vi "CRYRub & Buzz FFT.vi"(11 "wave data":dbl[](array[numeric])) -> (0 "Fe[n,kf]":dbl[][](array[numeric]), 1 "size":i32, 2 "Frame number":i32, 3 "F[k]":dbl[](array[numeric]))   [LabVIEW 2013]
uses:
  <vilib>/Analysis/2dsp.llb/Real FFT.vi
  <vilib>/Analysis/NI_AALPro.lvlib
  <vilib>/measure/NI_MABase.lvlib
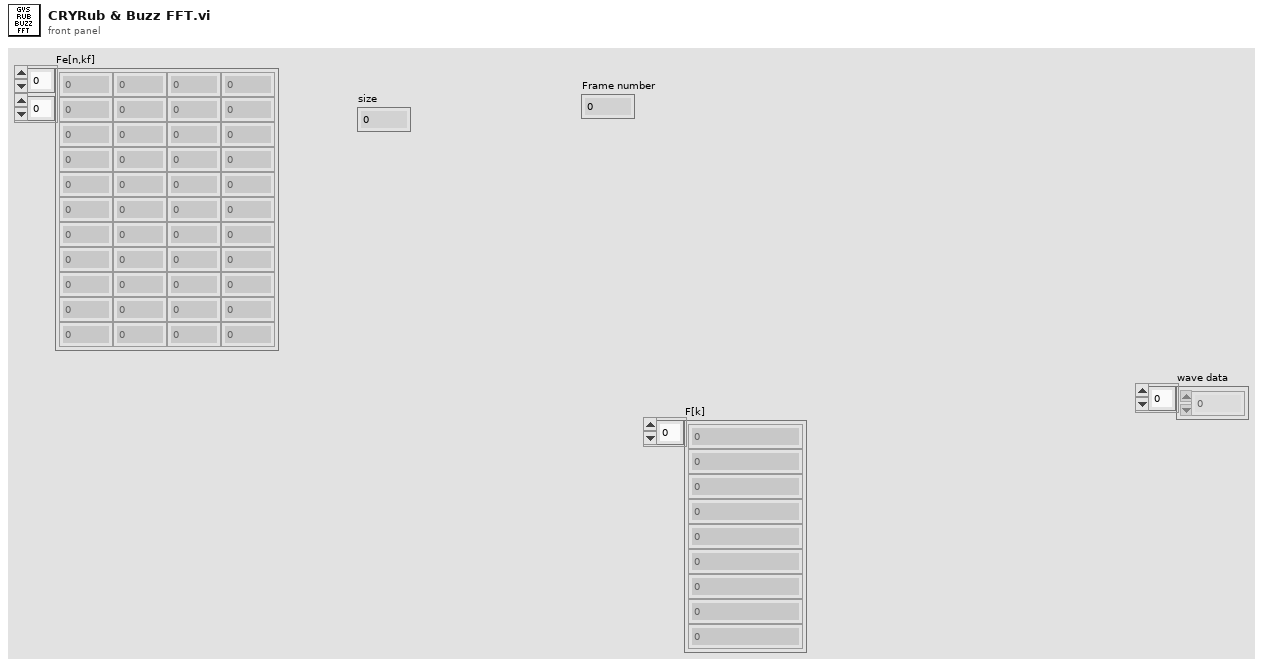
[diagram p1: front panel]
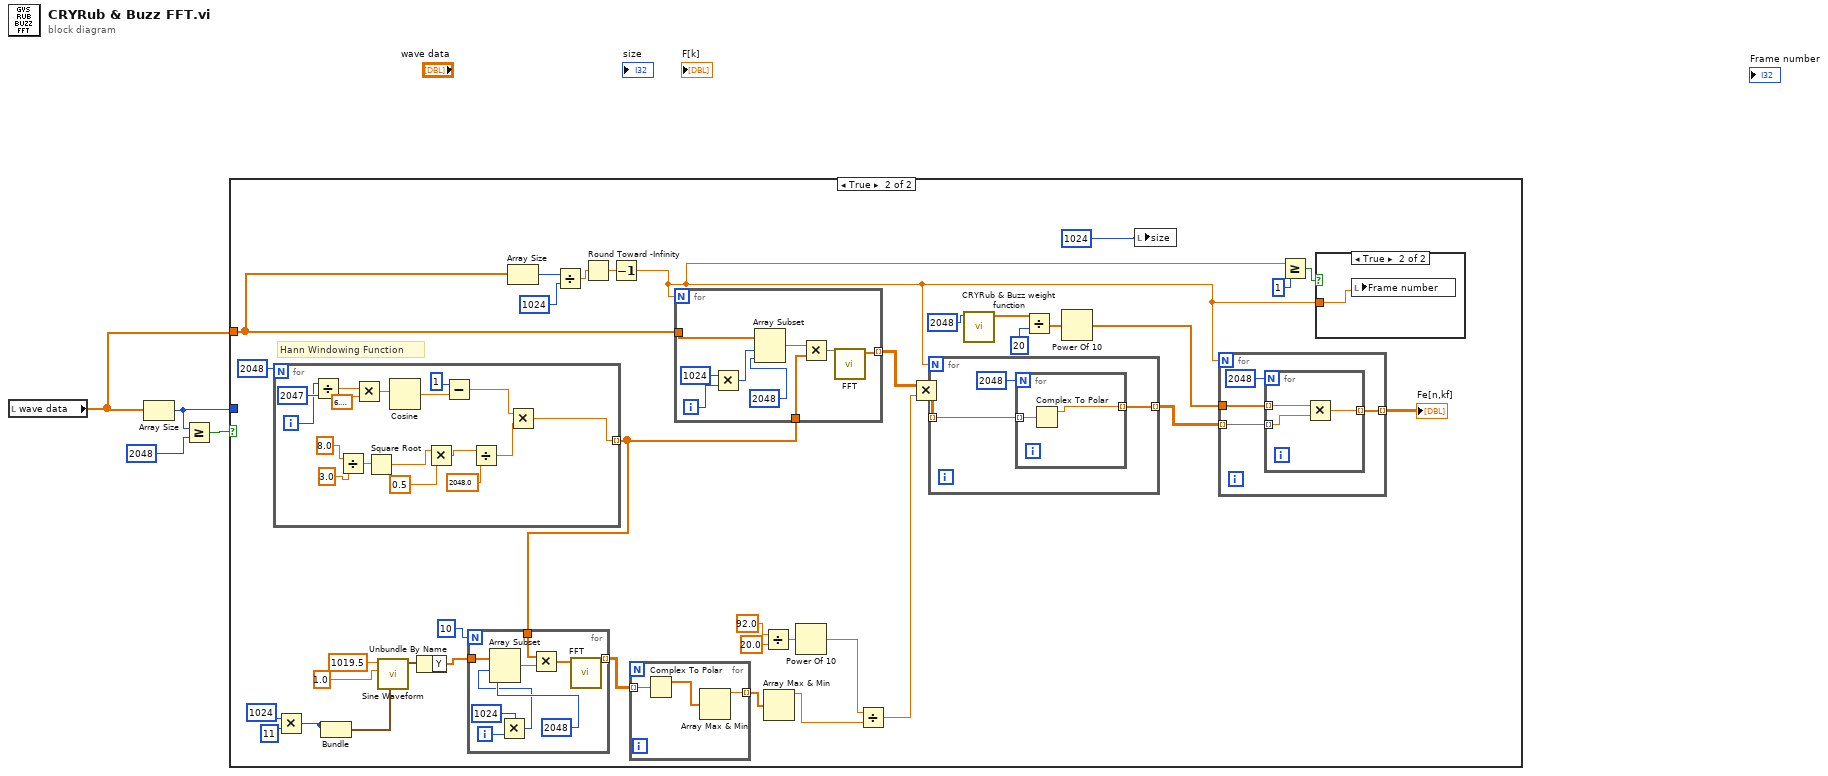
[diagram p0: block diagram]
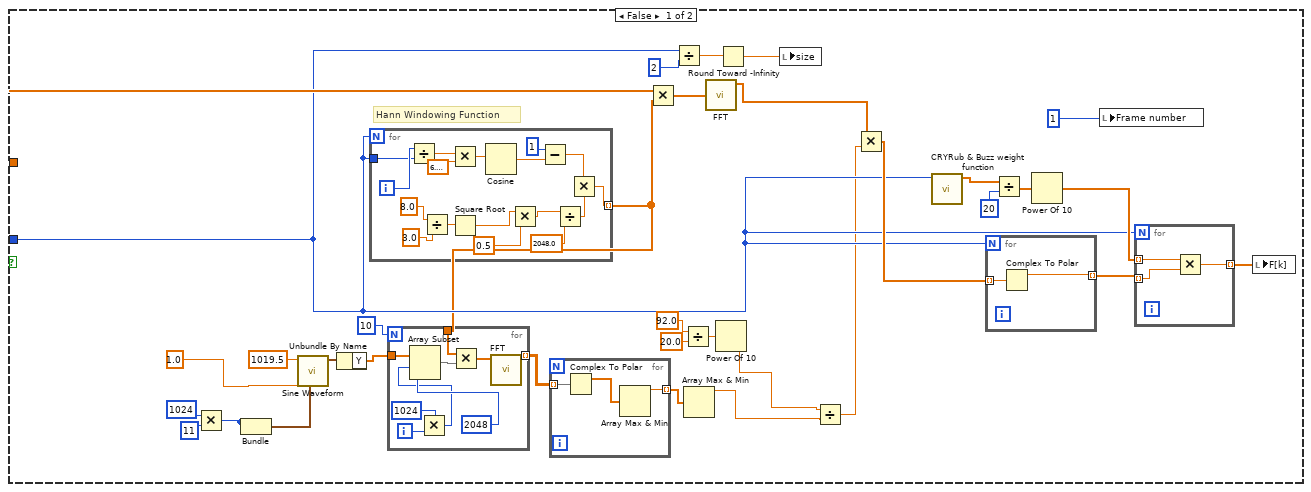
[diagram p2: hidden frame]
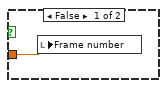
[diagram p3: hidden frame]
diagram:
  n1 = local read "wave data"() -> (w2:dbl[])
  n2 = Array Size(array=w2) -> (size(s)=w1:i32)
  n3 = Greater Or Equal?(x=w1, y=2048) -> (x >= y?=w3:bool)
  n4 = case shown="True" w3 {
    tunnel: w2 -> [w28 w97]
    tunnel: w1 -> [w23 _]
    frame False {
      # "Hann Windowing Function"
      n5 = Multiply(x=1024 ("length"), y=11) -> (x*y=w17:i32)
      n6 = Bundle(w17, w17) -> (w18:cluster{i32, i32})  [unwired: 1 in]
      n7 = call <vilib>:"Sine Waveform.vi"("sampling info"=w18, "amplitude"=1.0, "frequency"=1019.5) -> ("signal out"=w21:waveform(dbl))  [unwired: 7 in, 1 out]
      n8 = Unbundle By Name(w21) -> ("Y"=w16:dbl[])
      n9 = for {
        N: w23 -> [_]
        tunnel: [w50] -> w5 mode=indexing
        tunnel: w23 -> [w60]
        i -> [w61]
        n10 = Divide(x=w61, y=w60) -> (x/y=w64:dbl)
        n11 = Divide(x=8.0, y=3.0) -> (x/y=w56:dbl)
        n12 = Multiply(x=w64, y=6.283185307179586) -> (x*y=w65:dbl)
        n13 = Square Root(x=w56) -> (sqrt(x)=w55:dbl)
        n14 = Cosine(x=w65) -> (cos(x)=w66:dbl)
        n15 = Multiply(x=w55, y=0.5) -> (x*y=w54:dbl)
        n16 = Subtract(x=1, y=w66) -> (x-y=w52:dbl)
        n17 = Divide(x=w54, y=2048.0) -> (x/y=w51:dbl)
        n18 = Multiply(x=w52, y=w51) -> (x*y=w50:dbl)
      }
      n19 = for {
        N: 10 -> [_]
        tunnel: w16 -> [w42]
        tunnel: [w46] -> w15 mode=indexing
        tunnel: w5 -> [w40]
        i -> [w44]
        n20 = Multiply(x=1024 ("length"), y=w44) -> (x*y=w41:i32)
        n21 = Array Subset(array=w42, index=w41, length=2048) -> (w39:dbl[])
        n22 = Multiply(x=w40, y=w39) -> (x*y=w38:dbl[])
        n23 = call-poly <vilib>:"FFT.vi"("X"=w38) -> ("FFT {X}"=w46:cdb[])  [unwired: 9 in, 1 out]
      }
      n24 = for {
        tunnel: w15 -> [w49] mode=indexing
        tunnel: [w47] -> w13 mode=indexing
        n25 = Complex To Polar(r * e^(i*theta)=w49) -> (r=w48:dbl[])  [unwired: 1 out]
        n26 = Array Max & Min(array=w48) -> (max value=w47:dbl)  [unwired: 3 out]
      }
      n27 = Multiply(x=w28, y=w5) -> (x*y=w35:dbl[])
      n28 = Divide(x=w23, y=2) -> (x/y=w26:dbl)
      n29 = Divide(x=92.0, y=20.0) -> (x/y=w10:dbl)
      n30 = Array Max & Min(array=w13) -> (max value=w7:dbl)  [unwired: 3 out]
      n31 = call-poly <vilib>:"FFT.vi"("X"=w35) -> ("FFT {X}"=w34:cdb[])  [unwired: 9 in, 1 out]
      n32 = Power Of 10(x=w10) -> (10^x=w8:dbl)
      n33 = Round Toward -Infinity(1:w26) -> (0:w25:dbl)
      n34 = local write "size"(w25) -> ()
      n35 = Divide(x=w8, y=w7) -> (x/y=w6:dbl)
      n36 = Multiply(x=w34, y=w6) -> (x*y=w31:cdb[])
      n37 = call "CRYRub & Buzz weight function.vi"("Numeric"=w23) -> ("ear wight"=w37:dbl[])  [unwired: 9 in]
      n38 = for {
        N: w23 -> [_]
        tunnel: w31 -> [w71] mode=indexing
        tunnel: [w70] -> w32 mode=indexing
        n39 = Complex To Polar(r * e^(i*theta)=w71) -> (r=w70:dbl)  [unwired: 1 out]
      }
      n40 = Divide(x=w37, y=20) -> (x/y=w30:dbl[])
      n41 = Power Of 10(x=w30) -> (10^x=w33:dbl[])
      n42 = local write "Frame number"(1) -> ()
      n43 = for {
        N: w23 -> [_]
        tunnel: w33 -> [w69] mode=indexing
        tunnel: w32 -> [w68] mode=indexing
        tunnel: [w67] -> w36 mode=indexing
        n44 = Multiply ("Multiply.vi")(x=w69, y=w68) -> (x*y=w67:dbl)
      }
      n45 = local write "F[k]"(w36) -> ()
    }
    frame True {
      # "Hann Windowing Function"
      n46 = for {
        N: 2048 -> [_]
        tunnel: [w144] -> w74 mode=indexing
        i -> [w154]
        n47 = Divide(x=w154, y=2047) -> (x/y=w157:dbl)
        n48 = Divide(x=8.0, y=3.0) -> (x/y=w150:dbl)
        n49 = Multiply(x=w157, y=6.283185307179586) -> (x*y=w159:dbl)
        n50 = Square Root(x=w150) -> (sqrt(x)=w149:dbl)
        n51 = Cosine(x=w159) -> (cos(x)=w160:dbl)
        n52 = Multiply(x=w149, y=0.5) -> (x*y=w148:dbl)
        n53 = Subtract(x=1, y=w160) -> (x-y=w146:dbl)
        n54 = Divide(x=w148, y=2048.0) -> (x/y=w145:dbl)
        n55 = Multiply(x=w146, y=w145) -> (x*y=w144:dbl)
      }
      n56 = Multiply(x=1024 ("length"), y=11) -> (x*y=w81:i32)
      n57 = Bundle(w81, w81) -> (w80:cluster{i32, i32})  [unwired: 1 in]
      n58 = call <vilib>:"Sine Waveform.vi"("sampling info"=w80, "amplitude"=1.0, "frequency"=1019.5) -> ("signal out"=w77:waveform(dbl))  [unwired: 7 in, 1 out]
      n59 = Unbundle By Name(w77) -> ("Y"=w82:dbl[])
      n60 = for {
        N: 10 -> [_]
        tunnel: w82 -> [w113]
        tunnel: [w117] -> w83 mode=indexing
        tunnel: w74 -> [w111]
        i -> [w115]
        n61 = Multiply(x=1024 ("length"), y=w115) -> (x*y=w112:i32)
        n62 = Array Subset(array=w113, index=w112, length=2048) -> (w110:dbl[])
        n63 = Multiply(x=w111, y=w110) -> (x*y=w109:dbl[])
        n64 = call-poly <vilib>:"FFT.vi"("X"=w109) -> ("FFT {X}"=w117:cdb[])  [unwired: 9 in, 1 out]
      }
      n65 = Array Size(array=w97) -> (size(s)=w107:i32)
      n66 = Divide(x=w107, y=1024) -> (x/y=w105:dbl)
      n67 = Round Toward -Infinity(1:w105) -> (0:w101:dbl)
      n68 = Decrement(x=w101) -> (x-1=w72:dbl)
      n69 = for {
        tunnel: w83 -> [w120] mode=indexing
        tunnel: [w118] -> w85 mode=indexing
        n70 = Complex To Polar(r * e^(i*theta)=w120) -> (r=w119:dbl[])  [unwired: 1 out]
        n71 = Array Max & Min(array=w119) -> (max value=w118:dbl)  [unwired: 3 out]
      }
      n72 = for {
        N: w72 -> [_]
        tunnel: w97 -> [w141]
        tunnel: w74 -> [w135]
        tunnel: [w136] -> w104 mode=indexing
        i -> [w143]
        n73 = Multiply(x=1024, y=w143) -> (x*y=w140:i32)
        n74 = Array Subset(array=w141, index=w140, length=2048) -> (w137:dbl[])
        n75 = Multiply(x=w137, y=w135) -> (x*y=w138:dbl[])
        n76 = call-poly <vilib>:"FFT.vi"("X"=w138) -> ("FFT {X}"=w136:cdb[])  [unwired: 9 in, 1 out]
      }
      n77 = Divide(x=92.0, y=20.0) -> (x/y=w88:dbl)
      n78 = Array Max & Min(array=w85) -> (max value=w91:dbl)  [unwired: 3 out]
      n79 = Power Of 10(x=w88) -> (10^x=w90:dbl)
      n80 = Divide(x=w90, y=w91) -> (x/y=w75:dbl)
      n81 = Multiply(x=w104, y=w75) -> (x*y=w100:cdb[][])
      n82 = for {
        N: w72 -> [_]
        tunnel: w100 -> [w131] mode=indexing
        tunnel: [w130] -> w99 mode=indexing
        n83 = for {
          N: 2048 -> [_]
          tunnel: w131 -> [w134] mode=indexing
          tunnel: [w133] -> w130 mode=indexing
          n84 = Complex To Polar(r * e^(i*theta)=w134) -> (r=w133:dbl)  [unwired: 1 out]
        }
      }
      n85 = call "CRYRub & Buzz weight function.vi"("Numeric"=2048) -> ("ear wight"=w92:dbl[])  [unwired: 9 in]
      n86 = Divide(x=w92, y=20) -> (x/y=w102:dbl[])
      n87 = Power Of 10(x=w102) -> (10^x=w98:dbl[])
      n88 = local write "size"(1024) -> ()
      n89 = for {
        N: w72 -> [_]
        tunnel: w99 -> [w124] mode=indexing
        tunnel: w98 -> [w126]
        tunnel: [w123] -> w73 mode=indexing
        n90 = for {
          N: 2048 -> [_]
          tunnel: w126 -> [w129] mode=indexing
          tunnel: w124 -> [w128] mode=indexing
          tunnel: [w127] -> w123 mode=indexing
          n91 = Multiply ("Multiply.vi")(x=w129, y=w128) -> (x*y=w127:dbl)
        }
      }
      "Fe[n,kf]" <- w73
      n92 = Greater Or Equal?(x=w72, y=1) -> (x >= y?=w93:bool)
      n93 = case shown="True" w93 {
        tunnel: w72 -> [w121 w122]
        frame False {
          n94 = local write "Frame number"(w121) -> ()
        }
        frame True {
          n95 = local write "Frame number"(w122) -> ()
        }
      }
    }
  }
